vi "Register for Events.vi"(8 "error in (no error)":errorcluster, 11 "Async Coms in":refnum<class "Async Coms.lvclass">) -> (0 "error out":errorcluster, 2 "Event Refnums":T1, 3 "Async Coms out":refnum<class "Async Coms.lvclass">)   [LabVIEW 2022 SP3, in "Async Coms.lvclass"]
uses:
  Async Coms.lvclass
  Process Actor/XY Controller/XY Stage Data Class/Events.ctl
  Process Actor/XY Controller/XY Stage Data Class/XY Position.ctl
  Process Actor/XY Controller/XY Stage Data Class/Moving.ctl
  Process Actor/XY Controller/XY Stage Data Class/Homed.ctl
  Process Actor/XY Controller/XY Stage Data Class/Acceleration.ctl
  Process Actor/XY Controller/XY Stage Data Class/Current Speed.ctl
  Process Actor/XY Controller/XY Stage Data Class/Speed.ctl
  Process Actor/Process Framework/Process State Data/Events.ctl
  Process Actor/Process Framework/Process State Data/Process State Data.lvclass
  Process Actor/XY Controller/XY Stage Data Class/XY Stage Data Class.lvclass
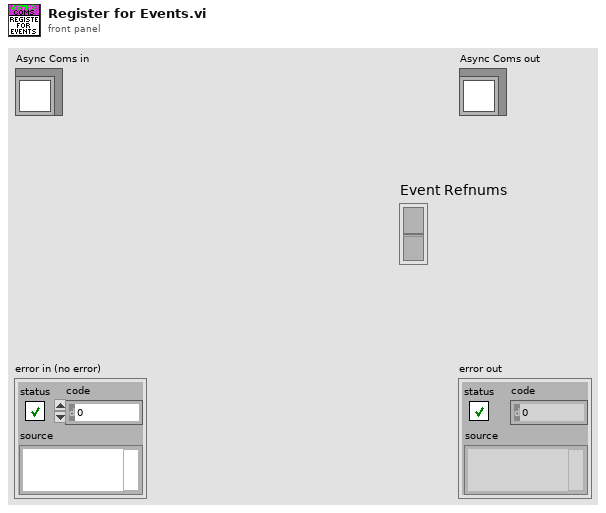
[diagram p1: front panel]
types:
  T1 = cluster{"Event Registration Refnum":refnum<event-registration>, "Event Registration Refnum":refnum<event-registration>}
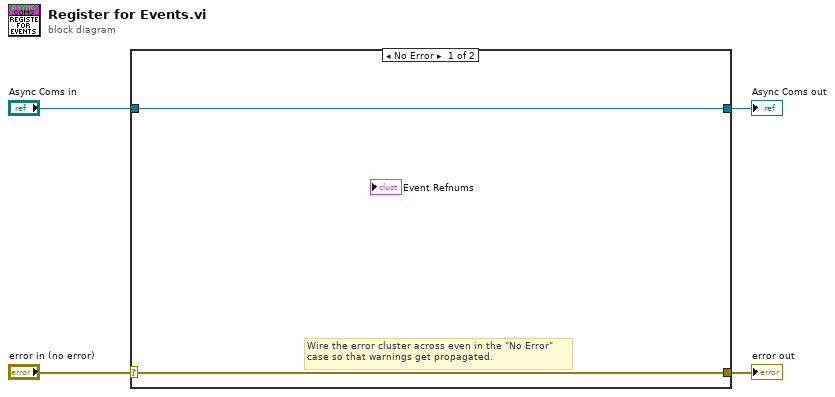
[diagram p0: block diagram]
diagram:
  n1 = case shown="No Error" "error in (no error)" {
    selector: "error in (no error)" -> [w5 w8]
    tunnel: [w5 w8] -> w3
    tunnel: [w6 w7] -> w1
    tunnel: "Async Coms in" -> [w6 w7]
    frame No Error {
      # "Wire the error cluster across even in the \"No Error\"\ncase so that warnings get propagated."
    }
    frame Error {
    }
  }
  "error out" <- w3
  "Async Coms out" <- w1
